vi "UI_Display.vi"(11 "AllControls In":T1) -> ()   [LabVIEW 2017]
uses:
  Ctrls/AllControls.ctl
  <vilib>/Utility/miscctls.llb/LVRowAndColumnTypeDef.ctl
  <vilib>/Utility/miscctls.llb/LVRowAndColumnUnsignedTypeDef.ctl
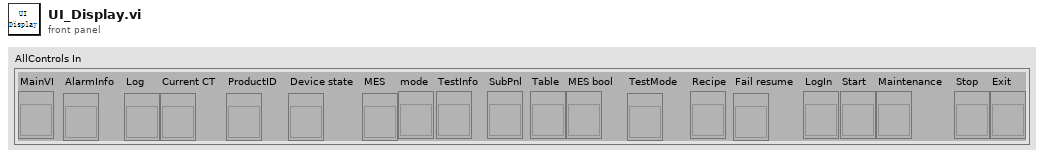
[diagram p1: front panel]
types:
  T1 = typedef "AllControls.ctl" = cluster{"MainVI":refnum<vi>, "AlarmInfo":refnum<vi>, "Log":refnum<vi>, "Current CT":refnum<vi>, "ProductID":refnum<vi>, "Device state":refnum<vi>, "MES":refnum<vi>, "mode":refnum<vi>, "TestInfo":refnum<vi>, "SubPnl":refnum<vi>, "Table":refnum<vi>, "MES bool":refnum<vi>, "TestMode":refnum<vi>, "Recipe":refnum<vi>, "Fail resume":refnum<vi>, "LogIn":refnum<vi>, "Start":refnum<vi>, "Maintenance":refnum<vi>, "Stop":refnum<vi>, "Exit":refnum<vi>}
  T2 = typedef "amc_Message Queue.ctl" = refnum<queue>
  T3 = cluster{"Vaule":string, "result":bool, "Step":i32}
  T4 = enum8{"Enabled", "Disabled", "Disabled and Grayed Out"}
  T5 = typedef "LVRowAndColumnTypeDef.ctl" = cluster{"Row":i32, "Column":i32}
  T6 = typedef "LVRowAndColumnUnsignedTypeDef.ctl" = cluster{"Row":u32, "Column":u32}
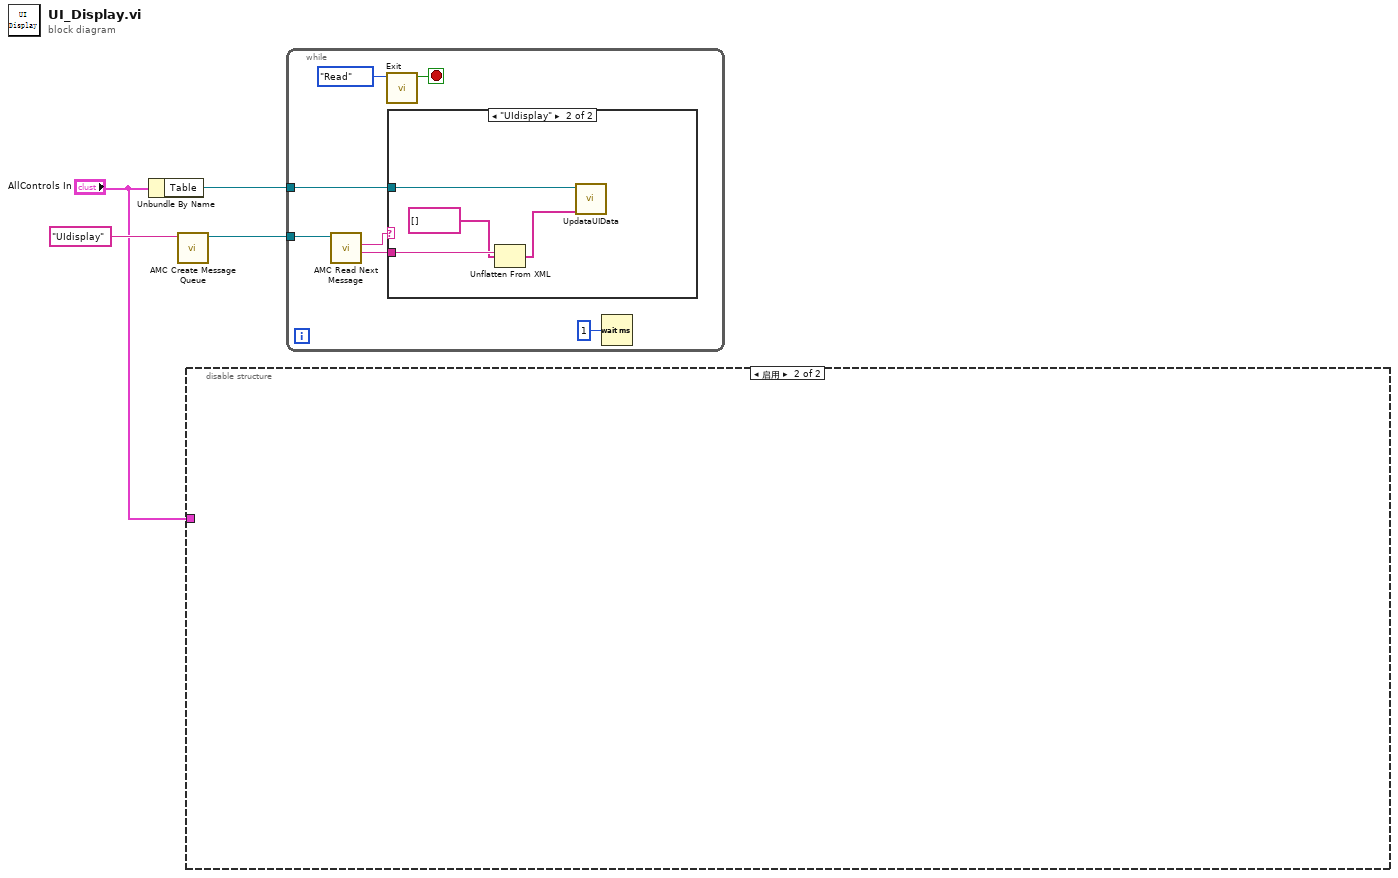
[diagram p0: block diagram]
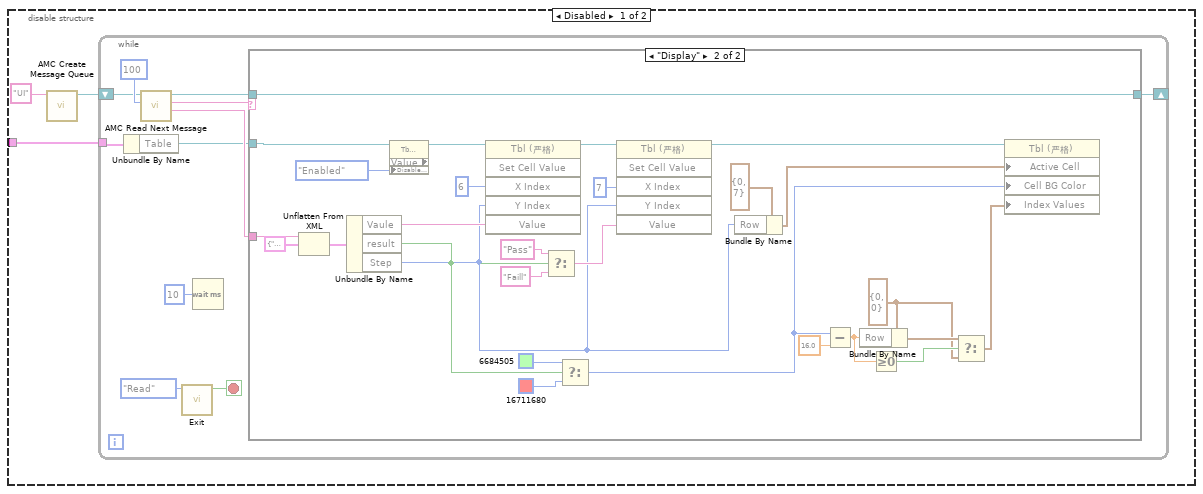
[diagram p2: hidden frame]
diagram:
  n1 = Unbundle By Name("AllControls In") -> ("Table"=w4:refnum<vi>)
  n2 = call "AMC Create Message Queue.vi"("Message Queue Name"="UIdisplay") -> ("Message Queue out"=w2:T2)  [unwired: 9 in, 1 out]
  n3 = disable-structure shown="启用" {
    disable-tunnel: "AllControls In" -> [w5 _]
    frame Disabled {
      n4 = call "AMC Create Message Queue.vi"("Message Queue Name"="UI" ("Message queue name (unnamed)")) -> ("Message Queue out"=w6:T2)  [unwired: 4 in, 6 out]
      n5 = while {
        shift-right: [w14] -> _
        shift-left: w6 -> [w16]
        tunnel: w5 -> [w12]
        stop <- w9 stop-if-true
        n6 = Unbundle By Name(w12) -> ("Table"=w10:refnum<vi>)
        n7 = call "AMC Read Next Message.vi"("timeout (1ms)"=100 ("Timeout"), "Message Queue in"=w16) -> ("Message Value"=w11:string, "Message Name"=w15:string, "Message Queue out"=w13:T2)  [unwired: 2 in, 5 out]
        n8 = call "Exit.vi"("Step"=enum16{"Initial", "Write", "Read"}."Read" ("step")) -> ("Exit Out"=w9:bool)  [unwired: 9 in, 1 out]
        n9 = Wait (ms)(milliseconds to wait=u32 10) -> ()  [unwired: 1 out]
        n10 = case shown="\"Display\"" w15 {
          tunnel: [w19 w47] -> w14
          tunnel: w13 -> [w19 w47]
          tunnel: w11 -> [_ w22]
          tunnel: w10 -> [_ w41]
          frame "假", Default {
          }
          frame "Display" {
            w26 = T6 {"Row"=0, "Column"=0} ("索引值")
            n11 = Unflatten From XML(xml string=w22, type=T3 {"Vaule"="", "result"=FALSE, "Step"=0} ("Vaule")) -> (value=w20:T3)  [unwired: 1 in, 1 out]
            n12 = Unbundle By Name(w20) -> ("Vaule"=w39:string, "result"=w32:bool, "Step"=w33:i32)
            n13 = property class="Tbl (严格)" props=["Value", "DisabledEnum"](reference=w41, "DisabledEnum"=T4."Enabled" ("禁用")) -> (reference out=w40:refnum<vi>)  [unwired: 1 in, 2 out]
            n14 = invoke class="Tbl (严格)" method="Set Cell Value"(reference=w40, "X Index"=6 ("Y索引"), "Y Index"=w33, "Value"=w39) -> (reference out=w46:refnum<vi>)  [unwired: 2 in, 5 out]
            n15 = Select(t="Pass", s=w32, f="Faill") -> (s? t:f=w36:string)
            n16 = Select(t=u32 6684505, s=w32, f=u32 16711680) -> (s? t:f=w24:u32)
            n17 = invoke class="Tbl (严格)" method="Set Cell Value"(reference=w46, "X Index"=7 ("Y索引"), "Y Index"=w33, "Value"=w36) -> (reference out=w43:refnum<vi>)  [unwired: 2 in, 5 out]
            n18 = Bundle By Name(cluster=T5 {"Row"=0, "Column"=7} ("活动单元格:活动单元格"), "Row"=w33) -> (w34:T5)
            n19 = Subtract(x=w24, y=16.0) -> (x-y=w28:dbl)
            n20 = Bundle By Name(cluster=w26, "Row"=w28) -> (w29:T6)
            n21 = Greater Or Equal To 0?(x=w28) -> (x >= 0?=w27:bool)
            n22 = Select(t=w29, s=w27, f=w26) -> (s? t:f=w23:T6)
            n23 = property class="Tbl (严格)"(reference=w43, "Active Cell"=w34, "Cell BG Color"=w24, "Index Values"=w23) -> ()  [unwired: 1 in, 2 out]
          }
        }
      }
    }
    frame Enabled {
    }
  }
  n24 = while {
    tunnel: w4 -> [w50]
    tunnel: w2 -> [w52]
    stop <- w53 stop-if-true
    n25 = call "AMC Read Next Message.vi"("Message Queue in"=w52) -> ("Message Value"=w49:string, "Message Name"=w51:string)  [unwired: 3 in, 6 out]
    n26 = call "Exit.vi"("Step"=enum16{"Initial", "Write", "Read"}."Read") -> ("Exit Out"=w53:bool)  [unwired: 9 in, 1 out]
    n27 = case shown="\"UIdisplay\"" w51 {
      tunnel: w50 -> [_ w58]
      tunnel: w49 -> [_ w57]
      frame "假", Default {
      }
      frame "UIdisplay" {
        n28 = Unflatten From XML(xml string=w57, type=string[] [] ("数组")) -> (value=w55:string[])  [unwired: 1 in, 1 out]
        n29 = call "UpdataUIData.vi"("数组"=w55, "表格输入"=w58) -> ()  [unwired: 10 in]
      }
    }
    n30 = Wait (ms)(milliseconds to wait=u32 1 ("等待时间（毫秒）")) -> ()  [unwired: 1 out]
  }
